vi "DAQmx_Read_better_performance.vi"() -> ()   [LabVIEW 2018]
uses:
  <vilib>/DAQmx/read.llb/DAQmx Read (Analog 1D DBL NChan 1Samp).vi
  <vilib>/DAQmx/create/channels.llb/DAQmx Create Channel (AI-Voltage-Basic).vi
  <vilib>/DAQmx/miscellaneous.llb/DAQmx Fill In Error Info.vi
panel:
  out "Average time per read":dbl
  out "data":dbl[][](array[numeric])
  in  "physical channels":tag[](array[tag])=["9207/ai0", "9207/ai1", "9207/ai2", "9207/ai3", "9207/ai4", "9207/ai5", "9207/ai6", "9207/ai7"]
  out "reading done":u32
  out "creation start":u32
  out "creation done":u32
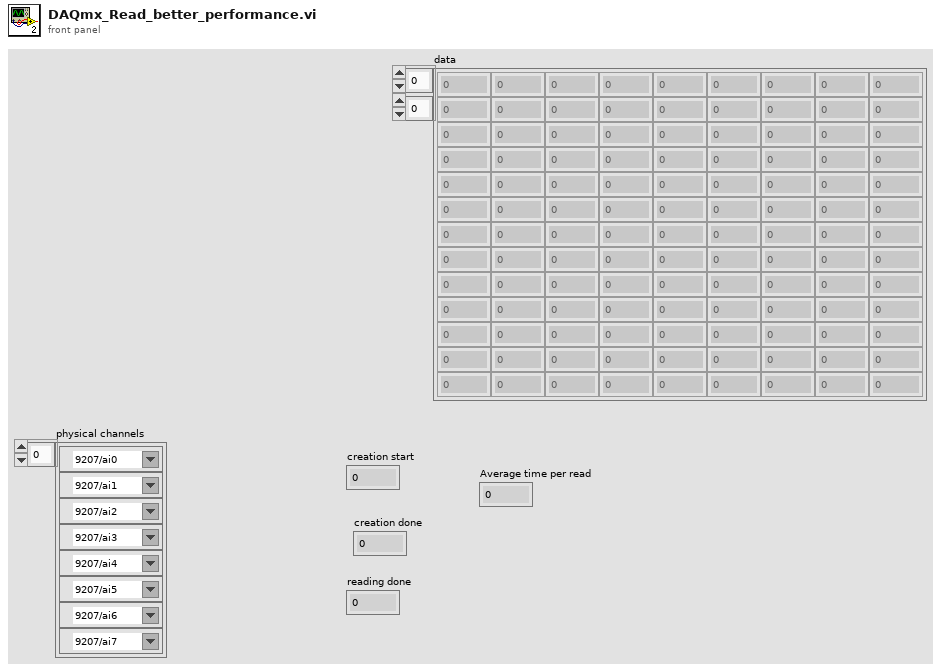
[diagram p1: front panel]
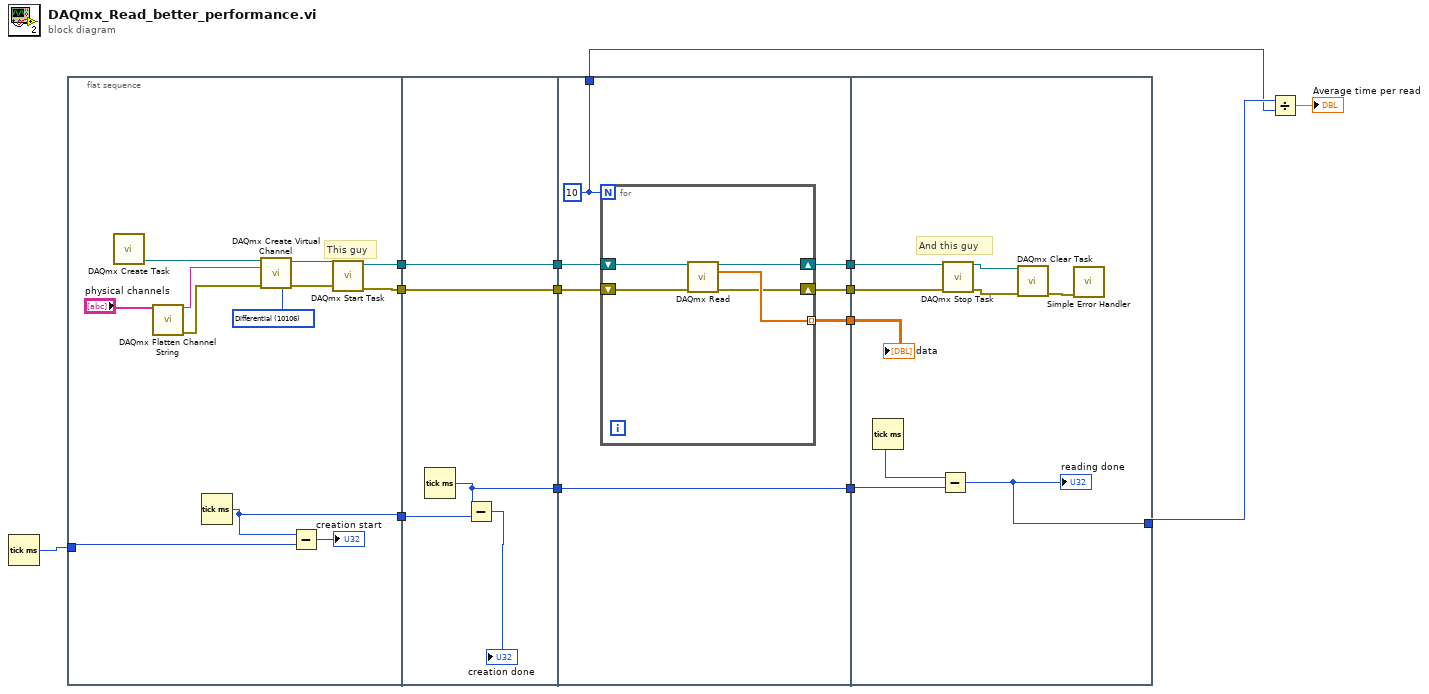
[diagram p0: block diagram]
diagram:
  n1 = Tick Count (ms)() -> (millisecond timer value=w14:u32)
  n2 = flat-sequence {
    tunnel: [w16] -> w13
    tunnel: [w15] -> w11
    tunnel: w14 -> [w25]
    tunnel: [w24] -> w9
    tunnel: w13 -> [w31]
    tunnel: [w31] -> w12
    tunnel: w11 -> [w30]
    tunnel: [w30] -> w10
    tunnel: w9 -> [w29]
    tunnel: [w27] -> w8
    tunnel: w12 -> [w34]
    tunnel: w10 -> [w33]
    tunnel: w8 -> [w37]
    tunnel: [w38] -> w7
    tunnel: [w37] -> w6
    tunnel: [w36] -> w5
    tunnel: [w35] -> w4
    tunnel: [w32] -> w2
    tunnel: w7 -> [w45]
    tunnel: w6 -> [w51]
    tunnel: w5 -> [w49]
    tunnel: w4 -> [w48]
    tunnel: [w44] -> w3
    frame #0 {
      w26 = 10106 items=["Default"=-1, "RSE"=10083, "NRSE"=10078, "Differential"=10106, "Pseudodifferential"=12529] ("input terminal configuration")
      # "This guy"
      n3 = call <vilib>:"DAQmx Create Task.vi"() -> ("task out"=w22:refnum<k21>)  [unwired: 14 in, 1 out]
      n4 = call <vilib>:"DAQmx Flatten Channel String.vi"("names in"="physical channels") -> ("names out"=w20:string, "error out"=w19:errorcluster)  [unwired: 13 in]
      n5 = Tick Count (ms)() -> (millisecond timer value=w24:u32)
      n6 = call-poly <vilib>:"DAQmx Create Virtual Channel.vi"("task in"=w22, "input terminal configuration"=w26, "physical channels"=w20, "error in"=w19) -> ("task out"=w18:refnum<k21>, "error out"=w17:errorcluster)  [unwired: 10 in]
      n7 = Subtract(x=w24, y=w25) -> (x-y=→"creation start":u32)
      n8 = call <vilib>:"DAQmx Start Task.vi"("task/channels in"=w18, "error in"=w17) -> ("task out"=w16:refnum<k21>, "error out"=w15:errorcluster)  [unwired: 12 in]
    }
    frame #1 {
      n9 = Tick Count (ms)() -> (millisecond timer value=w27:u32)
      n10 = Subtract(x=w27, y=w29) -> (x-y=→"creation done":u32)
    }
    frame #2 {
      w32 = 10
      n11 = for {
        N: w32 -> [_]
        tunnel: [w43] -> w38 mode=indexing
        shift-right: [w42] -> w36
        shift-left: w34 -> [w40]
        shift-right: [w41] -> w35
        shift-left: w33 -> [w39]
        n12 = call-poly <vilib>:"DAQmx Read.vi"("task/channels in"=w40, "error in"=w39) -> ("task out"=w42:refnum<k21>, "data"=w43:dbl[], "error out"=w41:errorcluster)  [unwired: 11 in]
      }
    }
    frame #3 {
      # "And this guy"
      n13 = Tick Count (ms)() -> (millisecond timer value=w52:u32)
      n14 = Subtract(x=w52, y=w51) -> (x-y=w44:u32)
      "reading done" <- w44
      n15 = call <vilib>:"DAQmx Stop Task.vi"("task/channels in"=w49, "error in"=w48) -> ("task out"=w47:refnum<k21>, "error out"=w46:errorcluster)  [unwired: 12 in]
      n16 = call <vilib>:"DAQmx Clear Task.vi"("task in"=w47, "error in"=w46) -> ("error out"=w50:errorcluster)  [unwired: 13 in]
      n17 = call <vilib>:"Simple Error Handler.vi"("error in (no error)"=w50) -> ()  [unwired: 4 in, 5 out]
      "data" <- w45
    }
  }
  n18 = Divide(x=w3, y=w2) -> (x/y=→"Average time per read":dbl)
